vi "Build Project Build Spec.vi"(0 "NSIS Installer":refnum<class "NSIS Installer.lvclass">, 11 "error IO":errorcluster) -> (4 "NSIS Installer":refnum<class "NSIS Installer.lvclass">, 15 "error out":errorcluster)   [LabVIEW 2017, in "CL_G3_VIComponentBuilder.lvlib" / "NSIS Installer.lvclass"]
doc: "Automates interaction with the NSIS installer builder."
uses:
  NSIS Installer.lvclass
  C:/builds/Component BuilderBT/SrcDist/Exports/Exports/Export.lvclass
  Exports/Export.lvclass/Export.ctl
  Exports/Accessors/Write Built Export's Full Path.vi
  Exports/Accessors/Read Exported Build Specification Path.vi
  Exports/Accessors/Read Export Operation Errors.vi
  <vilib>/Utility/file.llb/Is Path and Not Empty.vi
  <vilib>/Utility/libraryn.llb/Check if File or Folder Exists.vi
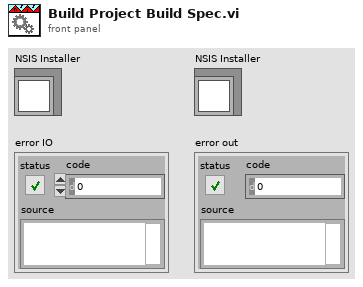
[diagram p1: front panel]
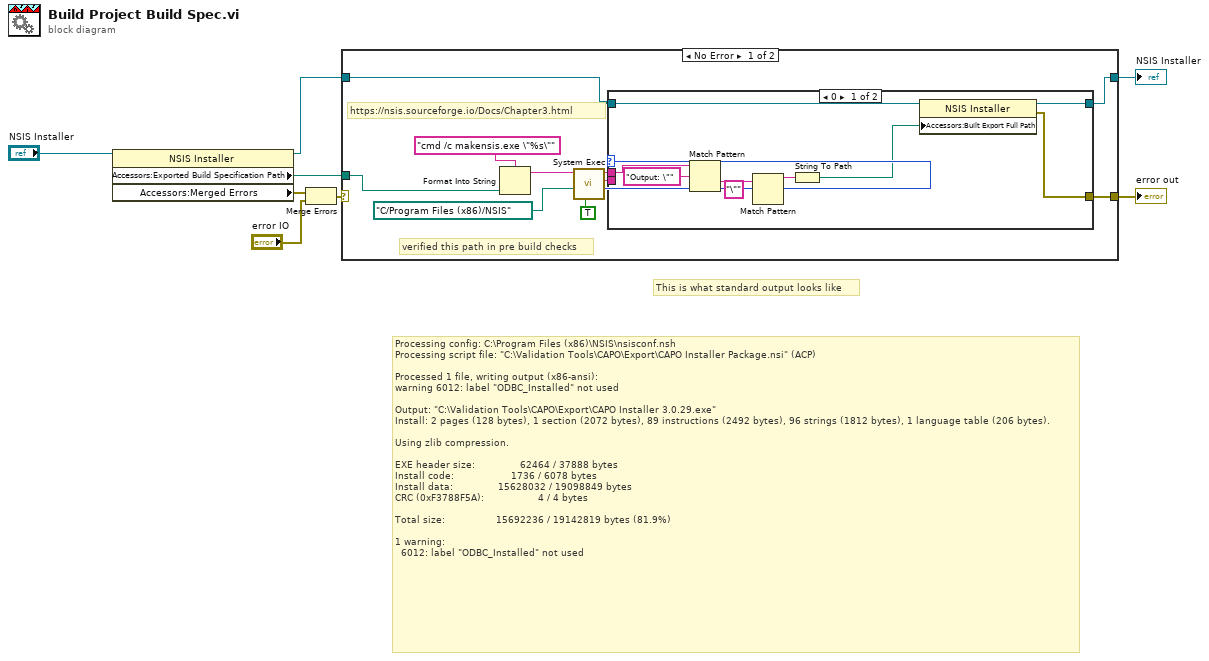
[diagram p0: block diagram]
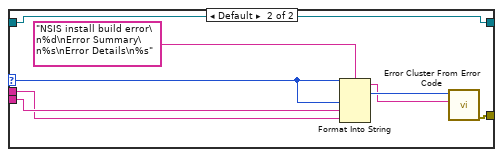
[diagram p2: hidden frame]
diagram:
  # "This is what standard output looks like"
  # "Processing config: C:\\Program Files (x86)\\NSIS\\nsisconf.nsh\nProcessing script file: \"C:\\Validation Tools\\CAPO\\Export\\CAPO Installer Package.nsi\" (ACP)\n\nProcessed 1 file, writing output (x86-ansi):\nwarning 6012: label \"ODBC_Installed\" not used\n\nOutput: \"C:\\Validation Tools\\CAPO\\Export\\CAPO Installer 3.0.29.exe\"\nInstall: 2 pages (128 bytes), 1 section (2072 bytes), 89 instructions (2492 bytes), 96 strings (1812 bytes), 1 language table (206 bytes).\n\nUsing zlib compression.\n\nEXE header size:               62464 / 37888 bytes\nInstall code:                   1736 / 6078 bytes\nInstall data:               15628032 / 19098849 bytes\nCRC (0xF3788F5A):                  4 / 4 bytes\n\nTotal size:                 15692236 / 19142819 bytes (81.9%)\n\n1 warning:\n  6012: label \"ODBC_Installed\" not used"
  n1 = property class="NSIS Installer"(reference="NSIS Installer") -> (reference out=w1:refnum<class "NSIS Installer.lvclass">, "Accessors:Exported Build Specification Path"=w7:path, "Accessors:Merged Errors"=w6:errorcluster)  [unwired: 1 in, 1 out]
  n2 = Merge Errors(w6, "error IO") -> (w4:errorcluster)
  n3 = case shown="No Error" w4 {
    selector: w4 -> [_ w37]
    tunnel: [w13 w37] -> w8
    tunnel: w1 -> [w10 w36]
    tunnel: w7 -> [w16 _]
    tunnel: [w9 w36] -> w3
    frame No Error {
      # "verified this path in pre build checks"
      # "https://nsis.sourceforge.io/Docs/Chapter3.html"
      n4 = Format Into String(format string="cmd /c makensis.exe \"%s\"", w16) -> (resulting string=w19:string)  [unwired: 2 in, 1 out]
      n5 = call <vilib>:"System Exec.vi"("run minimized? (F)"=TRUE, "working directory"=path "C:/Program Files (x86)/NSIS", "command line"=w19) -> ("return code"=w15:i32, "standard error"=w14:string, "standard output"=w12:string)  [unwired: 5 in, 1 out]
      n6 = case shown="0" w15 {
        selector: w15 -> [_ w33]
        tunnel: w14 -> [_ w32]
        tunnel: [w20 w35] -> w13
        tunnel: w12 -> [w26 w31]
        tunnel: w10 -> [w28 w29]
        tunnel: [w27 w29] -> w9
        frame 0 {
          n7 = Match Pattern(string=w26, regular expression="Output: \"") -> (after substring=w24:string)  [unwired: 1 in, 3 out]
          n8 = Match Pattern(string=w24, regular expression="\"") -> (before substring=w22:string)  [unwired: 1 in, 3 out]
          n9 = String To Path(string=w22) -> (path=w21:path)
          n10 = property class="NSIS Installer"(reference=w28, "Accessors:Built Export Full Path"=w21) -> (reference out=w27:refnum<class "NSIS Installer.lvclass">, error out=w20:errorcluster)  [unwired: 1 in]
        }
        frame Default {
          n11 = Format Into String(format string="NSIS install build error\n%d\nError Summary\n%s\nError Details\n%s", w33, w32, w31) -> (resulting string=w30:string)  [unwired: 2 in, 1 out]
          n12 = call <vilib>:"Error Cluster From Error Code.vi"("error message (\"\")"=w30, "error code (0)"=w33) -> ("error out"=w35:errorcluster)  [unwired: 7 in]
        }
      }
    }
    frame Error {
    }
  }
  "NSIS Installer" <- w3
  "error out" <- w8
